vi "plot.vi"(11 "Course":T2(array[cluster])) -> (3 "Image":T1(plugin-control))   [LabVIEW 2015]
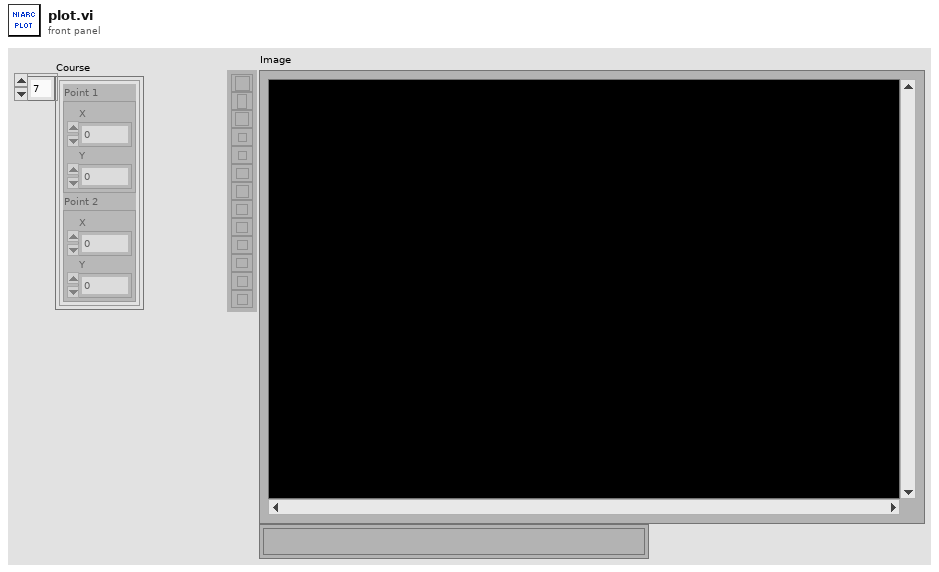
[diagram p1: front panel]
types:
  T1 = typedef "IMAQ Image.ctl" = refnum<image>
  T2 = cluster{"Point 1":cluster{"X":sgl, "Y":sgl}, "Point 2":cluster{"X":sgl, "Y":sgl}}[]
  T3 = cluster{"Left":i32, "Top":i32, "Right":i32, "Bottom":i32}
  T4 = cluster{"Point 1":cluster{"X":sgl, "Y":sgl}, "Point 2":cluster{"X":sgl, "Y":sgl}}
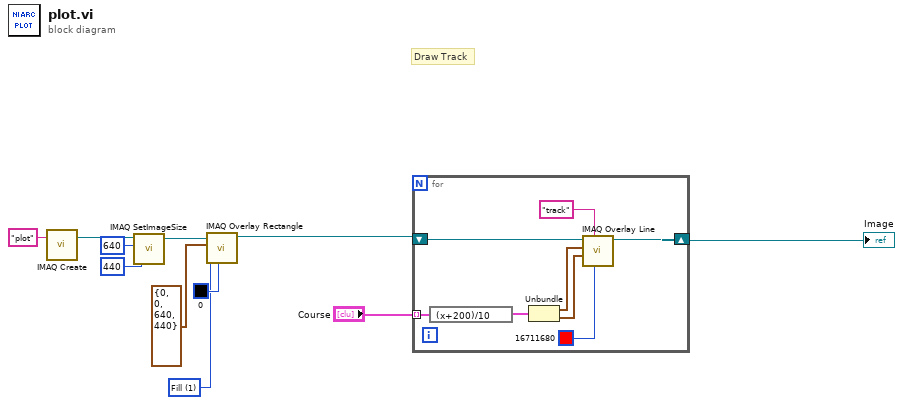
[diagram p0: block diagram]
diagram:
  w2 = u32 1 items=["Frame", "Fill", "Highlight"] ("Drawing Mode (Frame)")
  # "Draw Track"
  n1 = call "IMAQ Create"("Image Name"="plot") -> ("New Image"=w10:T1)  [unwired: 4 in, 1 out]
  n2 = call "IMAQ SetImageSize"("Y Resolution"=440, "X Resolution"=640, "Image"=w10) -> ("Image Out"=w6:T1)  [unwired: 2 in, 1 out]
  n3 = call "IMAQ Overlay Rectangle"("Color"=u32 0, "Drawing Mode (Frame)"=w2, "Rectangle"=T3 {"Left"=0, "Top"=0, "Right"=640, "Bottom"=440}, "Image"=w6) -> ("Image Out"=w4:T1)  [unwired: 6 in, 1 out]
  n4 = for {
    tunnel: "Course" -> [w15] mode=indexing
    shift-right: [w17] -> w1
    shift-left: w4 -> [w16]
    n5 = expression code="(x+200)/10"(w15) -> (w14:T4)
    n6 = Unbundle(w14) -> ("Point 1"=w13:cluster{"X":sgl, "Y":sgl}, "Point 2"=w12:cluster{"X":sgl, "Y":sgl})
    n7 = call "IMAQ Overlay Line"("Color"=u32 16711680, "Group"="track", "End Point"=w12, "Start Point"=w13, "Image"=w16) -> ("Image Out"=w17:T1)  [unwired: 5 in, 1 out]
  }
  "Image" <- w1
